vi "createChannels.vi"(8 "error in (no error)":errorcluster, 11 "niDAQmxDO in":refnum<class "niDAQmxDO.lvclass">) -> (0 "error out":errorcluster, 3 "niDAQmxDO out":refnum<class "niDAQmxDO.lvclass">)   [LabVIEW 2009, in "Hardware.lvlib" / "Channels.lvlib" / "niDAQmxDO.lvclass"]
uses:
  niDAQmxDO.lvclass
  <vilib>/DAQmx/create/channels.llb/DAQmx Create Channel (DO-Digital Output).vi
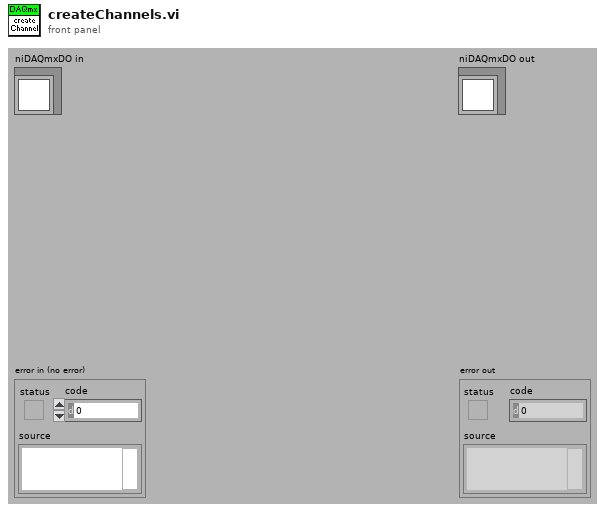
[diagram p1: front panel]
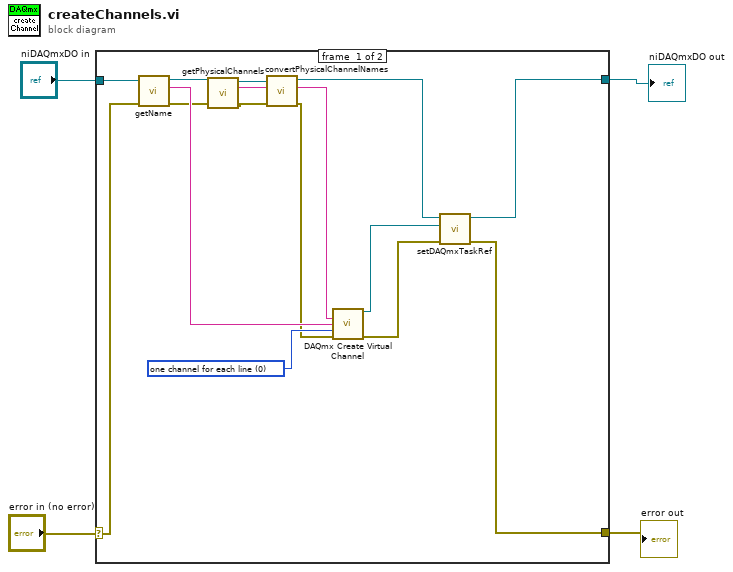
[diagram p0: block diagram]
diagram:
  n1 = case shown="No Error" "error in (no error)" {
    selector: "error in (no error)" -> [w19 w21]
    tunnel: "niDAQmxDO in" -> [w20 w22]
    tunnel: [w11 w22] -> w2
    tunnel: [w12 w21] -> w1
    frame #0 {
      w15 = 0 items=["one channel for each line", "one channel for all lines"] ("line grouping")
      n2 = call-dynamic "getName.vi"("error in (no error)"=w19, "DigitalOutput.lvclass in"=w20) -> ("error out"=w17:errorcluster, "name"=w18:string, "DigitalOutput.lvclass out"=w16:refnum<class "niDAQmxDO.lvclass">)  [unwired: 7 in]
      n3 = call-dynamic "getPhysicalChannels.vi"("error in (no error)"=w17, "DigitalOutput.lvclass in"=w16) -> ("error out"=w8:errorcluster, "Physical Channels"=w7:string, "DigitalOutput.lvclass out"=w10:refnum<class "niDAQmxDO.lvclass">)  [unwired: 7 in]
      n4 = call "convertPhysicalChannelNames.vi"("error in (no error)"=w8, "PhysicalChannels"=w7, "niDAQmxDO in"=w10) -> ("error out"=w6:errorcluster, "channel_names"=w5:string, "niDAQmxDO out"=w9:refnum<class "niDAQmxDO.lvclass">)  [unwired: 6 in]
      n5 = call-poly <vilib>:"DAQmx Create Virtual Channel.vi"("lines"=w5, "name to assign"=w18, "line grouping"=w15, "error in"=w6) -> ("task out"=w14:refnum<k21>, "error out"=w13:errorcluster)  [unwired: 10 in]
      n6 = call "setDAQmxTaskRef.vi"("error in (no error)"=w13, "DAQmx Task Ref"=w14, "niDAQmxDO.lvclass in"=w9) -> ("error out"=w12:errorcluster, "niDAQmxDO.lvclass out"=w11:refnum<class "niDAQmxDO.lvclass">)  [unwired: 7 in]
    }
    frame #1 {
    }
  }
  "error out" <- w1
  "niDAQmxDO out" <- w2
